vi "multicolumn listbox sort.vi"(4 "error IN":errorcluster, 6 "Bool Refnum":refnum<vi>, 7 "MCListbox Refnum":refnum<vi>) -> (0 "error out":errorcluster)   [LabVIEW 2015]
doc: "This VI sorts a multicolumn listbox when you click a column header. Click a column hearder once to sort that column in ascending order. Click the header again to sort the column in descending order. The VI reorders all other columns to maintain row integrity. You can wire a multicolumn listbox control reference to this VI."
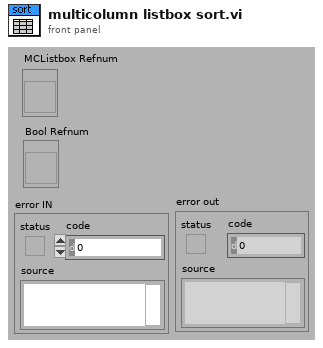
[diagram p1: front panel]
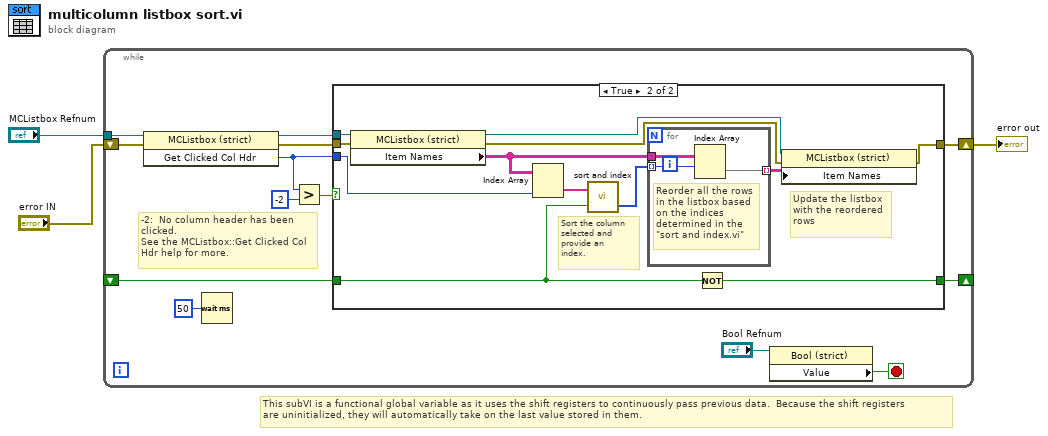
[diagram p0: block diagram]
diagram:
  # "This subVI is a functional global variable as it uses the shift registers to continuously pass previous data.  Because the shift registers \nare uninitialized, they will automatically take on the last value stored in them."
  n1 = while {
    shift-right: [w15] -> _
    shift-left: _ -> [w16]
    tunnel: "MCListbox Refnum" -> [w11]
    shift-right: [w6] -> w2
    shift-left: "error IN" -> [w7]
    stop <- w5 stop-if-true
    # "-2:  No column header has been       clicked.\nSee the MCListbox::Get Clicked Col Hdr help for more."
    n2 = invoke class="MCListbox (strict)" method="Get Clicked Col Hdr"(reference=w11, error in=w7) -> (reference out=w8:refnum<vi>, error out=w10:errorcluster, "Get Clicked Column Header"=w9:i32)  [unwired: 1 in]
    n3 = Wait (ms)(milliseconds to wait=u32 50) -> ()  [unwired: 1 out]
    n4 = Greater?(x=w9, y=-2) -> (0:w12:bool)
    n5 = case shown="True" w12 {
      tunnel: w9 -> [_ w30]
      tunnel: w16 -> [w18 w27]
      tunnel: [w18 w26] -> w15
      tunnel: w10 -> [w17 w24]
      tunnel: w8 -> [_ w25]
      tunnel: [w17 w19] -> w6
      frame False {
      }
      frame True {
        # "Update the listbox\nwith the reordered\nrows"
        # "Sort the column\nselected and provide an\nindex."
        n6 = property class="MCListbox (strict)"(reference=w25, error in=w24) -> (reference out=w20:refnum<vi>, error out=w21:errorcluster, "Item Names"=w23:string[][])
        n7 = Index Array(array=w23, index (col)=w30) -> (element=w29:string[])  [unwired: 1 in]
        n8 = call "sort and index.vi"("Reverse"=w27, "Array to Sort"=w29) -> ("Sorted Indices Array"=w28:i32[])  [unwired: 1 out]
        n9 = for {
          tunnel: w28 -> [w32] mode=indexing
          tunnel: w23 -> [w33]
          tunnel: [w31] -> w22 mode=indexing
          # "Reorder all the rows\nin the listbox based\non the indices determined in the \"sort and index.vi\""
          n10 = Index Array(array=w33, index (row)=w32) -> (element=w31:string[])  [unwired: 1 in]
        }
        n11 = Not(x=w27) -> (.not. x?=w26:bool)
        n12 = property class="MCListbox (strict)"(reference=w20, error in=w21, "Item Names"=w22) -> (error out=w19:errorcluster)  [unwired: 1 out]
      }
    }
    n13 = property class="Bool (strict)"(reference="Bool Refnum") -> ("Value"=w5:bool)  [unwired: 1 in, 2 out]
  }
  "error out" <- w2
